vi "Read Shared Library.vi"(8 "Error In":errorcluster, 11 "Session In":refnum<class "Session.lvclass">) -> (0 "Erorr Out":errorcluster, 2 "labssh2 Shared Library":path, 3 "Session Out":refnum<class "Session.lvclass">)   [LabVIEW 2017, in "LabSSH2.lvlib" / "Session.lvclass"]
uses:
  Session.lvclass
  Session.lvclass/Session.ctl
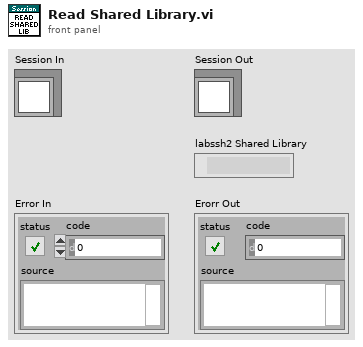
[diagram p1: front panel]
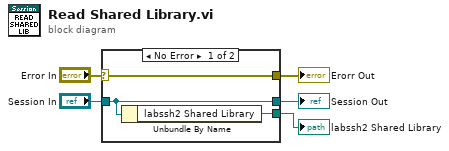
[diagram p0: block diagram]
diagram:
  n1 = case shown="No Error" "Error In" {
    selector: "Error In" -> [w8 w9]
    tunnel: [w8 w9] -> w4
    tunnel: "Session In" -> [w7 w10]
    tunnel: [w7 w10] -> w2
    tunnel: [w6 _] -> w1
    frame No Error {
      n2 = Unbundle By Name(w7) -> ("labssh2 Shared Library"=w6:path)
    }
    frame Error {
    }
  }
  "Erorr Out" <- w4
  "Session Out" <- w2
  "labssh2 Shared Library" <- w1
